vi "Experiment header-Write LOGIN section.vi"(8 "error in (no error)":errorcluster, 11 "Experiment header file ref":T1) -> (0 "error out":errorcluster, 3 "Experiment header file ref":T1)   [LabVIEW 2017]
uses:
  <vilib>/Utility/config.llb/Config Data RefNum.ctl
  User profiles code/Globals/gl_UsrProfiles globals.vi
  <vilib>/Utility/config.llb/Write Key (String).vi
  <vilib>/Utility/config.llb/NI_LVConfig.lvlib
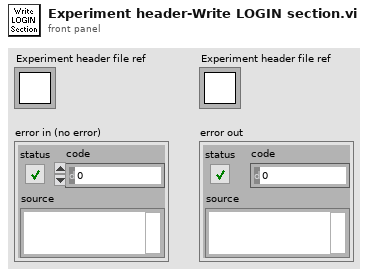
[diagram p1: front panel]
types:
  T1 = typedef "NI_LVConfig.lvlib/Config Data RefNum.ctl" = refnum<k1>
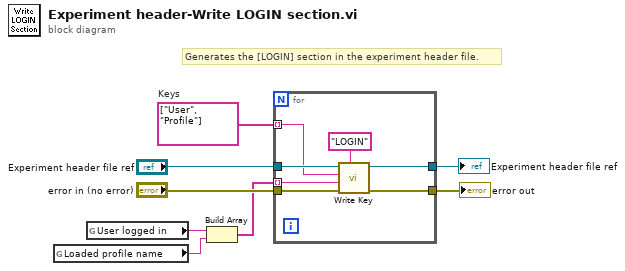
[diagram p0: block diagram]
diagram:
  w4 = string[] ["User", "Profile"]  # Keys
  # "Generates the [LOGIN] section in the experiment header file."
  n1 = global read "gl_UsrProfiles globals.vi" "Loaded profile name"() -> (w1:string)
  n2 = global read "gl_UsrProfiles globals.vi" "User logged in"() -> (w3:string)
  n3 = Build Array(w3, w1) -> (w2:string[])
  n4 = for {
    tunnel: [w15] -> w8
    tunnel: "error in (no error)" -> [w14]
    tunnel: [w13] -> w6
    tunnel: "Experiment header file ref" -> [w12]
    tunnel: w4 -> [w10] mode=indexing
    tunnel: w2 -> [w9] mode=indexing
    n5 = call-poly <vilib>:"Write Key.vi"("section"="LOGIN", "error in (no error)"=w14, "value"=w9, "key"=w10, "refnum"=w12) -> ("error out"=w15:errorcluster, "refnum out"=w13:T1)  [unwired: 4 in, 1 out]
  }
  "error out" <- w8
  "Experiment header file ref" <- w6
